vi "Read Test Recipe.vi"(6 "Base Path":path=path "C:/Test Recipes", 7 "Test Recipe in":refnum<class "Test Recipe.lvclass">, 8 "error in (no error)":errorcluster, 11 "Material Type":string) -> (0 "error out":errorcluster, 3 "Test Recipe out":refnum<class "Test Recipe.lvclass">)   [LabVIEW 2017, in "Test Recipe.lvlib" / "Test Recipe.lvclass"]
doc: "Reads a recipe for a specified Material Type and stores it into memory."
uses:
  Test Recipe.lvclass
  Test Recipe.lvclass/Test Recipe.ctl
  <vilib>/Utility/file.llb/Read Delimited Spreadsheet (string).vi
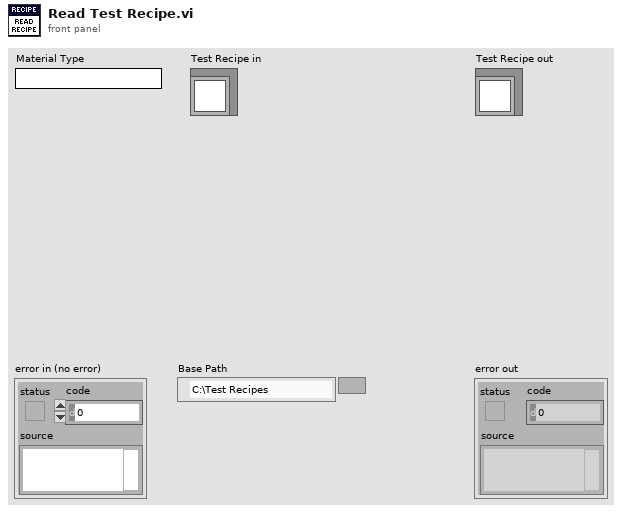
[diagram p1: front panel]
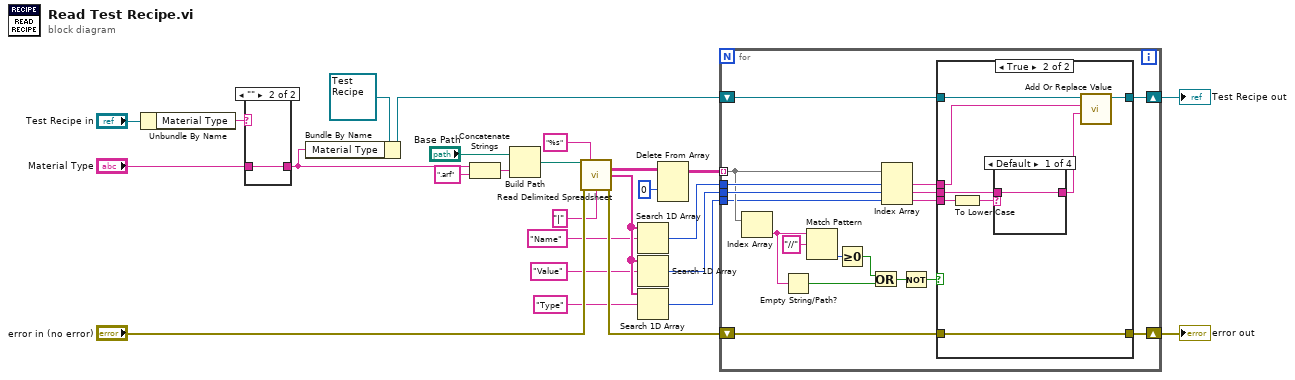
[diagram p0: block diagram]
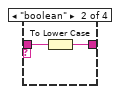
[diagram p4: hidden frame]
diagram:
  n1 = Unbundle By Name("Test Recipe in") -> ("Material Type"=w4:string)
  n2 = case shown="\"\"" w4 {
    selector: w4 -> [w27 _]
    tunnel: "Material Type" -> [_ w28]
    tunnel: [w27 w28] -> w1
    frame Default {
    }
    frame "" {
    }
  }
  n3 = Bundle By Name(cluster=refnum<class "Test Recipe.lvclass"> refnum ("Registry out"), "Material Type"=w1) -> (w2:refnum<class "Test Recipe.lvclass">)
  n4 = Concatenate Strings(w1, ".arf" ("string")) -> (w23:string)
  n5 = Build Path(base path="Base Path", name or relative path=w23) -> (appended path=w8:path)
  n6 = call-poly <vilib>:"Read Delimited Spreadsheet.vi"("file path (dialog if empty)"=w8, "format (%s)"="%s" ("format (%.3f)"), "error in (no error)"="error in (no error)", "delimiter (\\t)"="|" ("delimiter (\\t)")) -> ("all rows"=w14:string[][], "first row"=w20:string[], "error out"=w26:errorcluster)  [unwired: 6 in, 3 out]
  n7 = Search 1D Array(1D array=w20, element="Name") -> (index of element=w17:i32)  [unwired: 1 in]
  n8 = Search 1D Array(1D array=w20, element="Value") -> (index of element=w18:i32)  [unwired: 1 in]
  n9 = Search 1D Array(1D array=w20, element="Type") -> (index of element=w21:i32)  [unwired: 1 in]
  n10 = Delete From Array(array=w14, index (row)=0) -> (array with subset deleted=w16:string[][])  [unwired: 2 in, 1 out]
  n11 = for {
    tunnel: w16 -> [w44] mode=indexing
    tunnel: w17 -> [w46]
    tunnel: w18 -> [w45]
    shift-right: [w36] -> w9
    shift-left: w26 -> [w37]
    tunnel: w21 -> [w32]
    shift-right: [w29] -> w6
    shift-left: w2 -> [w30]
    n12 = Index Array(array=w44) -> (element=w42:string)  [unwired: 1 in]
    n13 = Empty String/Path?(string/path=w42) -> (empty?=w39:bool)
    n14 = Match Pattern(string=w42, regular expression="//") -> (offset past match=w40:i32)  [unwired: 1 in, 3 out]
    n15 = Greater Or Equal To 0?(x=w40) -> (x >= 0?=w38:bool)
    n16 = Or(x=w38, y=w39) -> (x .or. y?=w41:bool)
    n17 = Index Array(array=w44, index #1=w46, index #2=w45, index #3=w32) -> (element #1=w34:string, element #2=w33:string, element #3=w31:string)
    n18 = Not(x=w41) -> (.not. x?=w35:bool)
    n19 = case shown="True" w35 {
      tunnel: w37 -> [w48 w53]
      tunnel: [w48 w53] -> w36
      tunnel: w34 -> [_ w51]
      tunnel: w33 -> [_ w55]
      tunnel: w31 -> [_ w56]
      tunnel: w30 -> [w47 w52]
      tunnel: [w47 w49] -> w29
      frame False {
      }
      frame True {
        n20 = To Lower Case(string=w56) -> (all lower case string=w54:string)
        n21 = case shown="Default" w54 {
          tunnel: w55 -> [w57 w59 w60 w61]
          tunnel: [w57 w58 w60 w61] -> w50
          frame Default {
          }
          frame "boolean" {
            n22 = To Lower Case(string=w59) -> (all lower case string=w58:string)
          }
          frame "string" {
          }
          frame "decimal", "double", "integer", "numeric" {
          }
        }
        n23 = call-dynamic "Add Or Replace Value.vi"("Value"=w50, "Key"=w51, "Registry in"=w52) -> ("Registry out"=w49:refnum<class "Test Recipe.lvclass">)  [unwired: 6 in, 2 out]
      }
    }
  }
  "error out" <- w9
  "Test Recipe out" <- w6
